vi "PH_Sixpack.handle Reset.vi"(0 "VI in":refnum<vi>, 5 "error in (no error)":errorcluster) -> (14 "VI out":refnum<vi>, 19 "error out":errorcluster)   [LabVIEW 2014, in "PH_Sixpack.lvlib"]
doc: "Since the 6P's are reseted totally but not per axis only, all axes require a reconfiguration; therefore this is triggered by this VI."
uses:
  PH_Sixpack.lvlib
  PH_Basics/PH_Stepmotor_BaseClass/PH_Stepmotor_BaseClass.lvlib
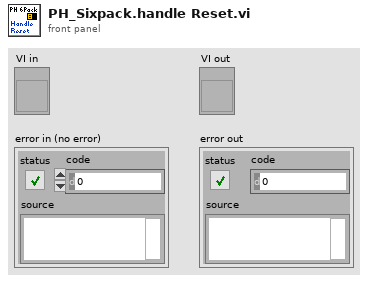
[diagram p1: front panel]
types:
  T1 = typedef "PH_Stepmotor_BaseClass.lvlib/PH_Stepmotor_BaseClass.i attribute.ctl" = cluster{"Device Error":errorcluster, "Axes PSDB Thread":cluster{"Ref":refnum<vi>, "Q-Ref":refnum<queue>, "Data Status":T2}, "Axes":T3[], "Axes PSDB Infos":cluster{"GUI Name":string, "PSDB Instance ID":i32, "PSDB Status Service ID":i32, "Axis":i32, "Class":string}[], "GUI Refs":T8}
  T2 = typedef "PH_PSDBWriter.lvlib/PH_PSDBWriter.Data Status.ctl" = i16
  T3 = typedef "PH_Stepmotor_BaseClass.lvlib/PH_Stepmotor_BaseClass.Axis Attributes.ctl" = cluster{"Settings":T4, "Endswitch?":bool, "DIM Service IDs":T6, "Activity":T7, "Configured?":bool, "Position":cluster{"Current":i32, "Target":i32}, "Position to set":cluster{"New?":bool, "Wanted":i32}, "Stop?":bool, "Reset?":bool, "Move?":bool, "Nothing connected?":bool}
  T4 = typedef "PH_Stepmotor_BaseClass.lvlib/PH_Stepmotor_BaseClass.Axis Settings.ctl" = cluster{"Sign change":bool, "Width":dbl, "Calibration":dbl, "Unit":string, "Motor Type":T5, "Unit Width":string, "Unit CF":string}
  T5 = typedef "PH_Stepmotor_BaseClass.lvlib/PH_Stepmotor_BaseClass.Motor Type.ctl" = enum16{"Unspecific", "OWIS 49.120.2633", "OWIS 49.060.1033", "OWIS 43.040.2558", "Diamond Motion 2200 series", "OWIS 49.120.266B.MV6", "Calorimeter", "Linear Stage 1", "MICOS VT-80", "MICOS VT-80 S", "Standa Rotstage nt0.95A", "PUF RA 320.200", "PUF RA 800.200", "PUF RA 800.400", "PUF RA 400.50", "1324.nn.800.50", "1324.n9c.800.50", "1324.nn.320.200", "1324.nn.400.200", "1324.nn.800.200", "1324.nn.400.50", "1324.8c9c.800.50", "1324.8c9c.400.200"}
  T6 = typedef "PH_Stepmotor_BaseClass.lvlib/PH_Stepmotor_BaseClass.Axis DIM Service IDs.ctl" = cluster{"Settings":i32, "Information":i32}
  T7 = typedef "PH_Stepmotor_BaseClass.lvlib/PH_Stepmotor_BaseClass.Axis Activity.ctl" = enum16{"No Information", "stopped", "running", "Failure", "Alarm", "stopped at backward ES", "stopped at foreward ES"}
  T8 = typedef "PH_Stepmotor_BaseClass.lvlib/PH_Stepmotor_BaseClass.GUI Refs.ctl" = cluster{"Axes Configuration":refnum<vi>, "Device Error":refnum<vi>, "Axes PSDB Infos":refnum<vi>}
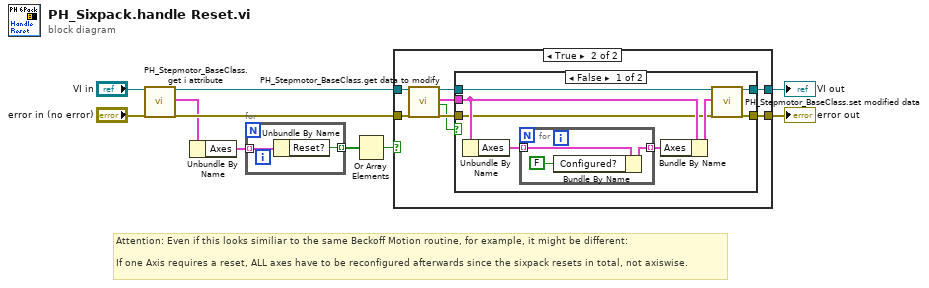
[diagram p0: block diagram]
diagram:
  # "Attention: Even if this looks similiar to the same Beckoff Motion routine, for example, it might be different:\n \nIf one Axis requires a reset, ALL axes have to be reconfigured afterwards since the sixpack resets in total, not axiswise."
  n1 = call "PH_Stepmotor_BaseClass.get i attribute.vi"("i ref in"="VI in", "error in (no error)"="error in (no error)") -> ("i ref out"=w4:refnum<vi>, "i attribute"=w7:T1, "error out"=w9:errorcluster)  [unwired: 15 in]
  n2 = Unbundle By Name(w7) -> ("Axes"=w6:T3[])
  n3 = for {
    tunnel: w6 -> [w12] mode=indexing
    tunnel: [w11] -> w5 mode=indexing
    n4 = Unbundle By Name(w12) -> ("Reset?"=w11:bool)
  }
  n5 = Or Array Elements(Boolean array=w5) -> (logical OR=w1:bool)
  n6 = case shown="True" w1 {
    tunnel: w9 -> [w13 w22]
    tunnel: w4 -> [w14 w21]
    tunnel: [w14 w19] -> w3
    tunnel: [w13 w16] -> w2
    frame False {
    }
    frame True {
      n7 = call "PH_Stepmotor_BaseClass.get data to modify.vi"("i ref in"=w21, "error in (no error)"=w22) -> ("i ref out"=w20:refnum<vi>, "i attribute"=w18:T1, "timed out"=w15:bool, "error out"=w17:errorcluster)  [unwired: 14 in]
      n8 = case shown="False" w15 {
        tunnel: w20 -> [w30 w35]
        tunnel: [w29 w35] -> w19
        tunnel: w18 -> [w27 _]
        tunnel: w17 -> [w24 w34]
        tunnel: [w23 w34] -> w16
        frame False {
          n9 = Unbundle By Name(w27) -> ("Axes"=w26:T3[])
          n10 = for {
            tunnel: w26 -> [w33] mode=indexing
            tunnel: [w32] -> w25 mode=indexing
            n11 = Bundle By Name(cluster=w33, "Configured?"=FALSE) -> (w32:T3)
          }
          n12 = Bundle By Name(cluster=w27, "Axes"=w25) -> (w28:T1)
          n13 = call "PH_Stepmotor_BaseClass.set modified data.vi"("i ref in"=w30, "i attribute"=w28, "error in (no error)"=w24) -> ("i ref out"=w29:refnum<vi>, "error out"=w23:errorcluster)  [unwired: 15 in]
        }
        frame True {
        }
      }
    }
  }
  "VI out" <- w3
  "error out" <- w2
